vi "Calculate surface Cp.vi"(2 "U_inf":sgl[](array[numeric])=[1.0, 0.0, 0.0], 3 "Panel triangles in":T1[](array[typedef])) -> (0 "Panel ctrl pts.":sgl[][](array[numeric]), 1 "Cp":sgl[](array[numeric]))   [LabVIEW 2017]
uses:
  ctls/Triangle panel.ctl
panel:
  out "i":i32(graph)
  # "PN 26/10/17"
  # "Vertices"
  # "Edges"
  # "Unit normal"
  # "Control point"
  # "Edge\nlinks \n(tri index)"
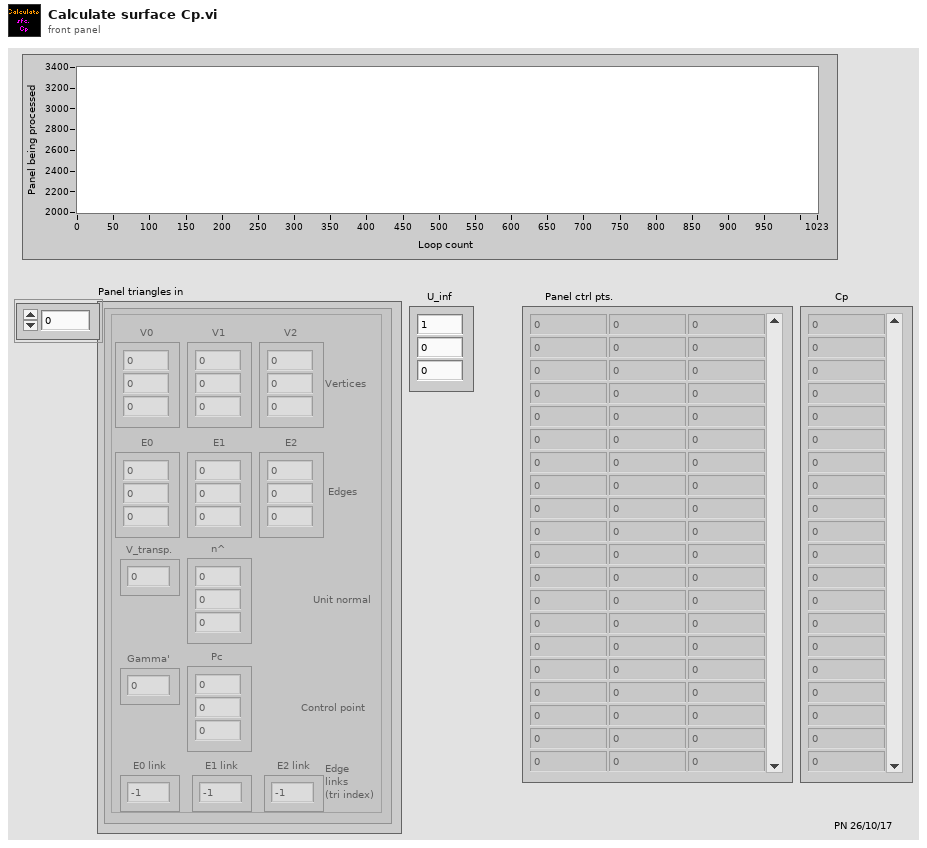
[diagram p1: front panel]
types:
  T1 = typedef "Triangle panel.ctl" = cluster{"V0":sgl[], "V1":sgl[], "V2":sgl[], "E0":sgl[], "E1":sgl[], "E2":sgl[], "n^":sgl[], "Pc":sgl[], "Gamma'":sgl, "V_transp.":sgl, "E0 link":i32, "E1 link":i32, "E2 link":i32}
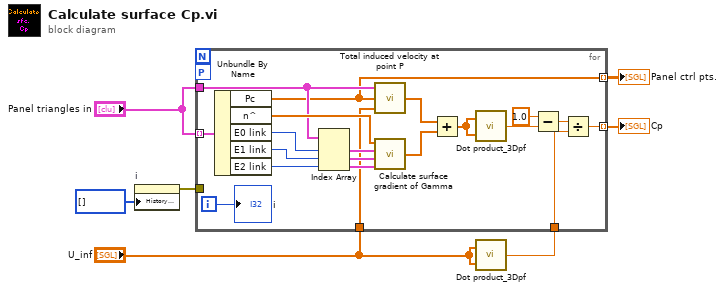
[diagram p0: block diagram]
diagram:
  n1 = property on="i" class="WFChart (strict)"("History Data"=i32[] []) -> (error out=w2:errorcluster)  [unwired: 2 in, 1 out]
  n2 = call "Dot product_3Dpf.vi"("B"="U_inf", "A"="U_inf") -> ("A . B"=w7:sgl)
  n3 = for {
    tunnel: "Panel triangles in" -> [w25]
    tunnel: "Panel triangles in" -> [w27] mode=indexing
    workers-P: _ -> [_]
    tunnel: w7 -> [w12]
    tunnel: [w11] -> w5 mode=indexing
    tunnel: "U_inf" -> [w10]
    tunnel: [w9] -> w4 mode=indexing
    tunnel: w2 -> [_]
    i -> [w8]
    n4 = Unbundle By Name(w27) -> ("Pc"=w9:sgl[], "n^"=w26:sgl[], "E0 link"=w24:i32, "E1 link"=w23:i32, "E2 link"=w22:i32)
    n5 = Index Array(array=w25, index #1=w24, index #2=w23, index #3=w22) -> (element #1=w21:T1, element #2=w20:T1, element #3=w19:T1)
    n6 = call "Total induced velocity at point P.vi"("U_inf"=w10, "P"=w9, "Triangle panels"=w25) -> ("(U, V, W) at P"=w18:sgl[])
    n7 = call "Calculate surface gradient of Gamma.vi"("Panel linked to E2"=w19, "Panel linked to E1"=w20, "Panel linked to E0"=w21, "Centre panel n^"=w26) -> ("0.5*Grad_s(Gamma)"=w17:sgl[])
    n8 = Add(x=w18, y=w17) -> (x+y=w16:sgl[])
    n9 = call "Dot product_3Dpf.vi"("B"=w16, "A"=w16) -> ("A . B"=w14:sgl)
    n10 = Subtract(x=sgl 1.0, y=w14) -> (x-y=w13:sgl)
    n11 = Divide(x=w13, y=w12) -> (x/y=w11:sgl)
    "i" <- w8
  }
  "Panel ctrl pts." <- w4
  "Cp" <- w5
